vi "Acquire Data.vi"(0 "Data in":cluster{"Data":sgl[][]}[](array[cluster]), 1 "Trigger Index":i32, 5 "taskID":u32, 7 "Device Channel Lists":T11(array[cluster]), 9 "CJTEMP Chan Indexes":T12(array[cluster]), 11 "Channel Filter":bool[](array[boolean])) -> (4 "Data out":cluster{"Data":sgl[][]}[](array[cluster]), 6 "Acquiring Data":bool, 15 "error out":errorcluster)   [LabVIEW 2019]
uses:
  AI Read (waveform).vi
  AI Read (scaled array).vi
  <vilib>/measure/NI_MAPro.lvlib
  <vilib>/measure/mamon.llb/Trigger Detection for 1 Channel (obs).vi
  Type Defs and Controls/DAQ Settings.ctl
  Type Defs and Controls/Channel Config.ctl
  Type Defs and Controls/Header.ctl
  Type Defs and Controls/Sensor Config.ctl
  Type Defs and Controls/Trigger Stop Method.ctl
  Type Defs and Controls/Log File Type.ctl
  Type Defs and Controls/Graph Settings Type Def.ctl
  Type Defs and Controls/Test Limits.ctl
  Type Defs and Controls/Part Info.ctl
  Type Defs and Controls/All Part Info.ctl
panel:
  in  "taskID in":u32 format="%x"
  out "DAQ Active":bool
  in  "Data In":sgl[][](array[numeric])
  out "Data Out":sgl[][](array[numeric])
  out "DAQ Active out":bool
  in  "DAQ Active in":bool=TRUE
  in  "Config":T1={"DAQ Settings"={"Trigger Type"=enum."Manual", "Trigger Samples"=0, "Pretrigger Samples"=0, "Trigger Interval"=0.0, "Time Units"=FALSE, "Auto Save"=FALSE, "Sample Rate"=7.0, "Select Analog"=FALSE, "Trigger Value"=0.0, "Trigger Stop Method"=enum."Use Samples Value to Stop Trigger", "Rate Sec/Min"=FALSE, "Save Mode"=enum."Single File", "File Size Limit"=0.0, "Log File Type"=enum."Basic", "Trigger Data Index"=0}, "Channels"=[], "Header"={"TA Number"="", "Test Name"="", "Serial Number"="", "Technician"=""}, "Graph Settings"={"Graph Labels"=[], [], [], [], [], [], [], [], [], [], [], [], [], "Graph Toggles"=[], "Axis Toggles"=[], "Graph Range"=enum."1"}, "Test Limits"=[], "All Type Info"=[], "Save Mode"=enum."Single File"} {"DAQ Settings"."Trigger Interval" min=0.0; "DAQ Settings"."Pretrigger Samples" min=0; "DAQ Settings"."Trigger Samples" min=0}
  out "Data":sgl[][](array[numeric])
  # "EGU"
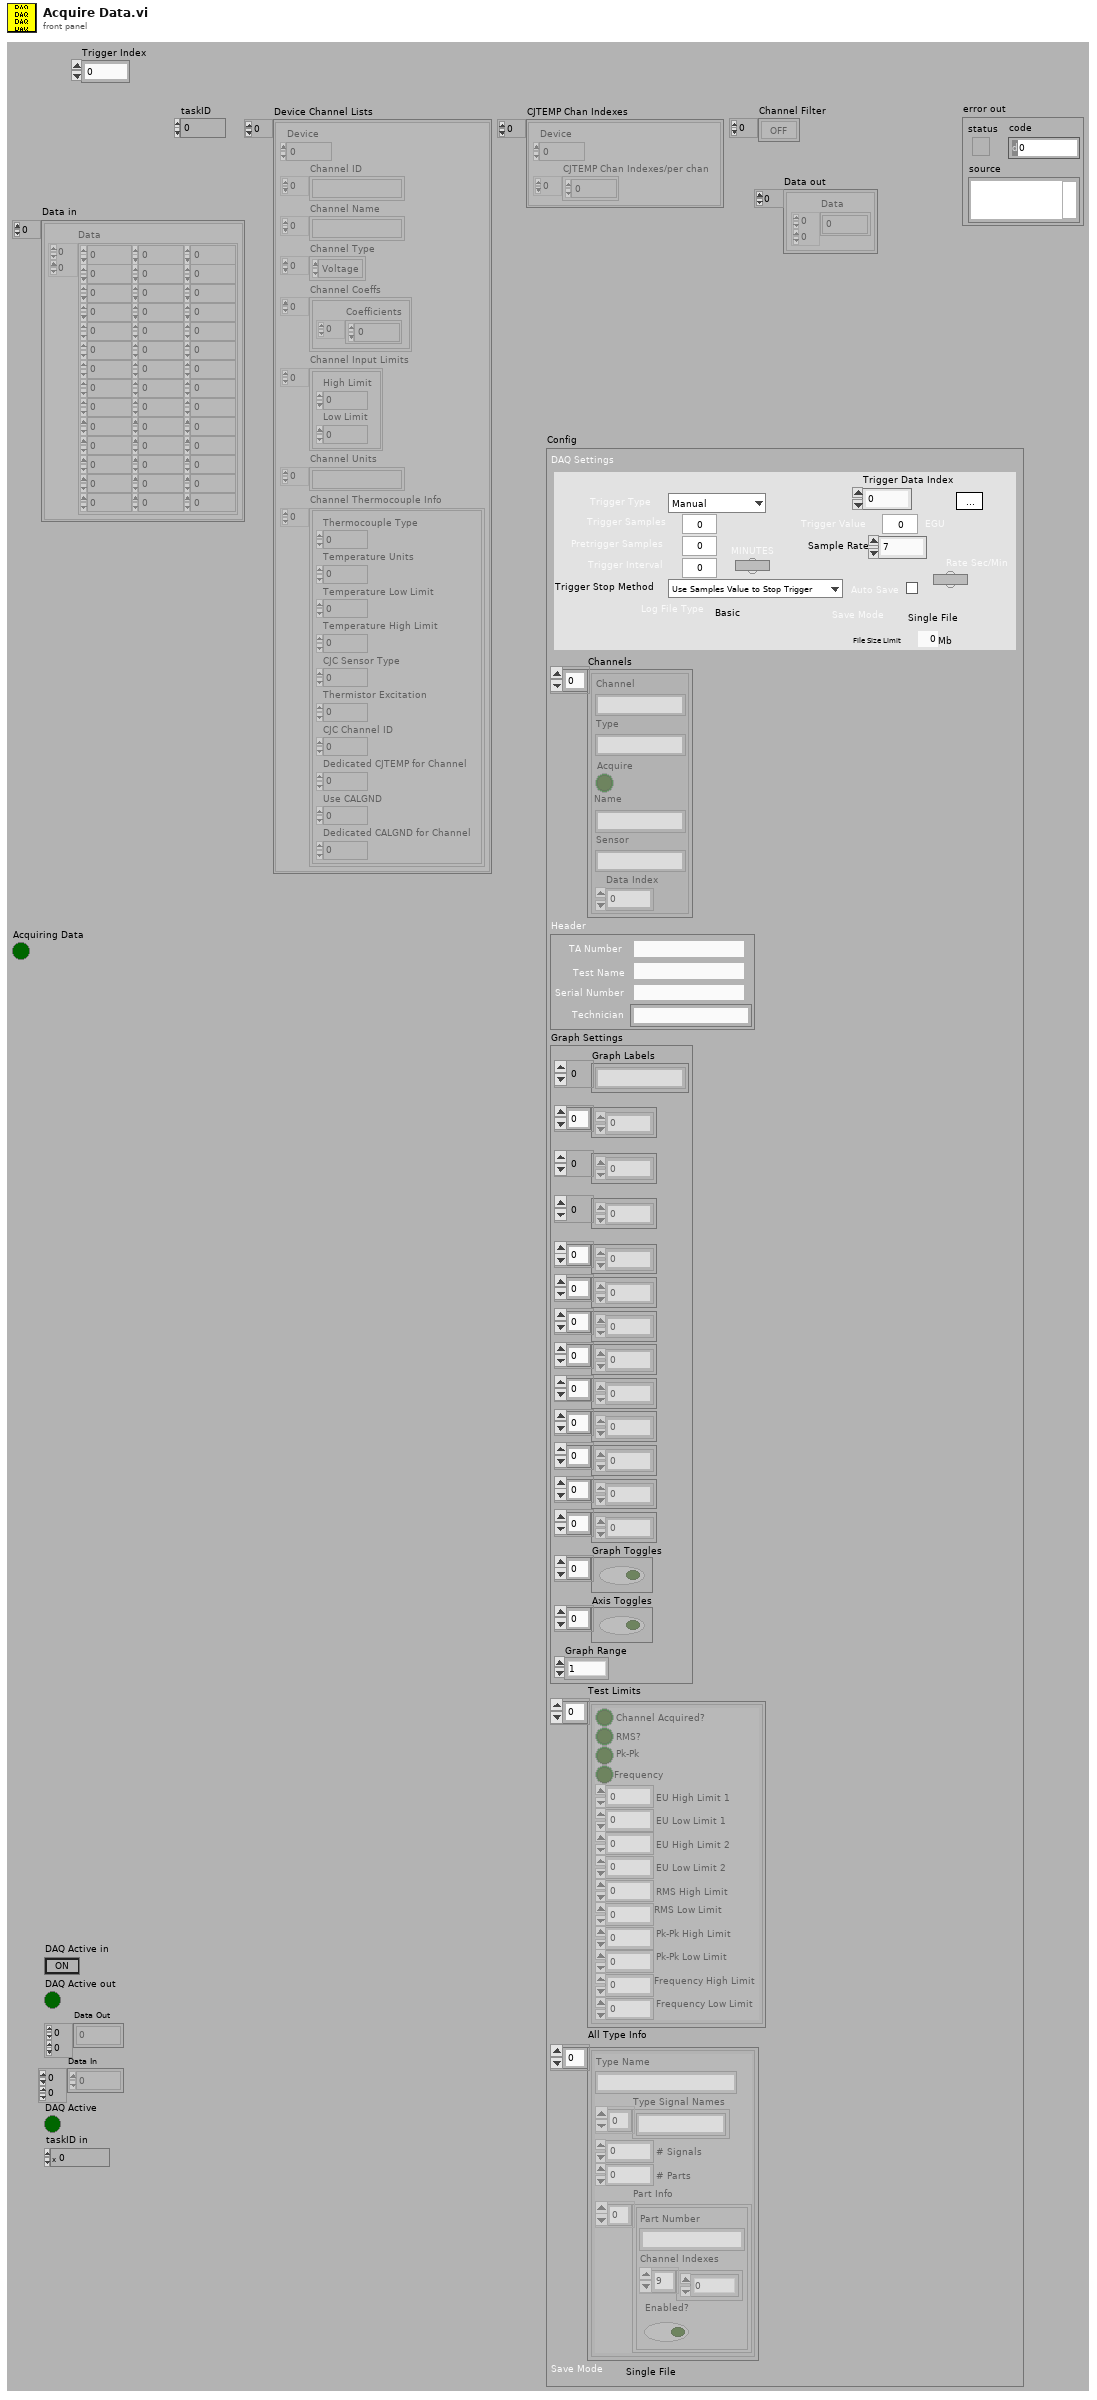
[diagram p1: front panel]
types:
  T1 = typedef "Sensor Config.ctl" = cluster{"DAQ Settings":T2, "Channels":T5[], "Header":T6, "Graph Settings":T7, "Test Limits":T8[], "All Type Info":T9, "Save Mode":enum16{"Single File", "Segmented Files", "New File at Midnight"}}
  T2 = typedef "DAQ Settings.ctl" = cluster{"Trigger Type":enum16{"Manual", "Timed", "Analog Rising", "Analog Falling"}, "Trigger Samples":i32, "Pretrigger Samples":i32, "Trigger Interval":dbl, "Time Units":bool, "Auto Save":bool, "Sample Rate":dbl, "Select Analog":bool, "Trigger Value":dbl, "Trigger Stop Method":T3, "Rate Sec/Min":bool, "Save Mode":enum16{"Single File", "Segmented Files", "New File at Midnight"}, "File Size Limit":dbl, "Log File Type":T4, "Trigger Data Index":u32}
  T3 = typedef "Trigger Stop Method.ctl" = enum16{"Use Samples Value to Stop Trigger", "Use Threshold to Stop Trigger"}
  T4 = typedef "Log File Type.ctl" = enum16{"Basic", "RTS"}
  T5 = typedef "Channel Config.ctl" = cluster{"Channel":string, "Type":string, "Acquire":bool, "Name":string, "Sensor":string, "Data Index":u32}
  T6 = typedef "Header.ctl" = cluster{"TA Number":string, "Test Name":string, "Serial Number":string, "Technician":string}
  T7 = typedef "Graph Settings Type Def.ctl" = cluster{"Graph Labels":string[], u8[], i16[], u32[], u8[], u8[], u8[], u32[], u8[], u8[], u8[], dbl[], dbl[], "Graph Toggles":bool[], "Axis Toggles":bool[], "Graph Range":enum16{"1", "2", "3", "4", "5", "10", "15", "30", "60"}}
  T8 = typedef "Test Limits.ctl" = cluster{"Channel Acquired?":bool, "RMS?":bool, "Pk-Pk":bool, "Frequency":bool, "EU High Limit 1":dbl, "EU Low Limit 1":dbl, "EU High Limit 2":dbl, "EU Low Limit 2":dbl, "RMS High Limit":dbl, "RMS Low Limit":dbl, "Pk-Pk High Limit ":dbl, "Pk-Pk Low Limit":dbl, "Frequency High Limit":dbl, "Frequency Low Limit":dbl}
  T9 = typedef "All Part Info.ctl" = cluster{"Type Name":string, "Type Signal Names":string[], "# Signals":i32, "# Parts":i32, "Part Info":T10[]}[]
  T10 = typedef "Part Info.ctl" = cluster{"Part Number":string, "Channel Indexes":u16[], "Enabled?":bool}
  T11 = cluster{"Device":i16, "Channel ID":string[], "Channel Name":string[], "Channel Type":enum16{"Voltage", "Thermocouple"}[], "Channel Coeffs":cluster{"Coefficients":dbl[]}[], "Channel Input Limits":cluster{"High Limit":dbl, "Low Limit":dbl}[], "Channel Units":string[], "Channel Thermocouple Info":cluster{"Thermocouple Type":u16, "Temperature Units":u16, "Temperature Low Limit":sgl, "Temperature High Limit":sgl, "CJC Sensor Type":u16, "Thermistor Excitation":u16, "CJC Channel ID":u16, "Dedicated CJTEMP for Channel":u16, "Use CALGND":u16, "Dedicated CALGND for Channel":u16}[]}[]
  T12 = cluster{"Device":i16, "CJTEMP Chan Indexes/per chan":i32[]}[]
  T13 = enum16{"Manual", "Timed", "Analog Rising", "Analog Falling"}
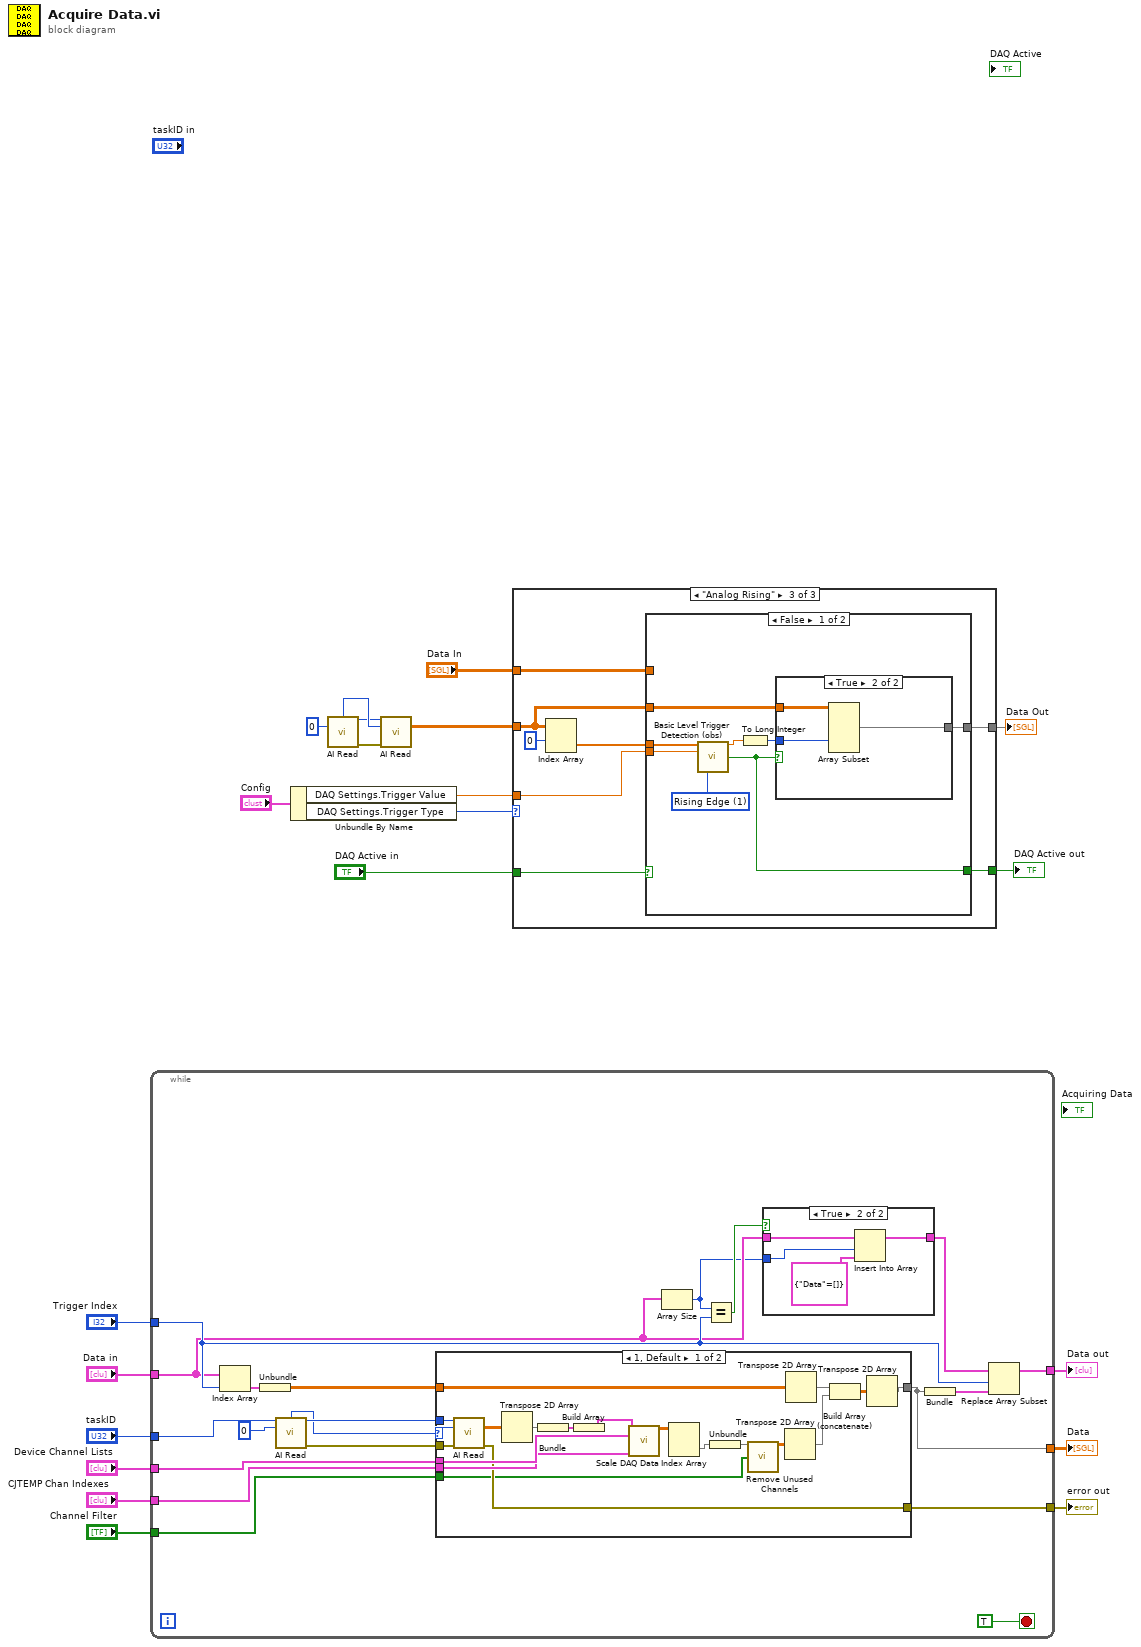
[diagram p0: block diagram]
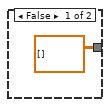
[diagram p4: hidden frame]
diagram:
  n1 = while {
    tunnel: [w41] -> w21
    tunnel: "Device Channel Lists" -> [w40]
    tunnel: "taskID" -> [w39]
    tunnel: "CJTEMP Chan Indexes" -> [w38]
    tunnel: "Channel Filter" -> [w37]
    tunnel: [w36] -> w16
    tunnel: [w35] -> w15
    tunnel: "Trigger Index" -> [w34]
    tunnel: "Data in" -> [w33]
    stop <- TRUE stop-if-true
    n2 = Index Array(array=w33, index=w34) -> (element=w29:cluster{"Data":sgl[][]})
    n3 = Unbundle(w29) -> ("Data"=w28:sgl[][])
    n4 = call-poly "AI Read.vi"("taskID in"=w39, "number of scans to read (-1:all)"=0) -> ("scan backlog"=w24:u32, "taskID out"=w30:u32, "error out"=w31:errorcluster)  [unwired: 8 in, 3 out]
    n5 = case shown="1, Default" w24 {
      selector: w24 -> [w57 _]
      tunnel: w30 -> [w66 _]
      tunnel: w31 -> [w65 _]
      tunnel: w40 -> [w61 _]
      tunnel: w38 -> [w60 _]
      tunnel: [w51 w67] -> w36
      tunnel: w28 -> [w54 w67]
      tunnel: [w56 _] -> w41
      tunnel: w37 -> [w47 _]
      frame 1, Default {
        n6 = call-poly "AI Read.vi"("taskID in"=w66, "number of scans to read (-1:all)"=w57, "error in (no error)"=w65) -> ("scaled data"=w64:sgl[][], "error out"=w56:errorcluster)  [unwired: 7 in, 4 out]
        n7 = Transpose 2D Array(2D array=w64) -> (transposed array=w50:sgl[][])
        n8 = Bundle(w50) -> (w63:cluster{sgl[][]})  [unwired: 1 in]
        n9 = Build Array(w63) -> (w62:cluster{sgl[][]}[])
        n10 = call "Scale DAQ Data.vi"("Data Read"=w62, "Coefficients"=w61, 11:w60) -> ("Scaled Data"=w59:sgl[][])  [unwired: 12 in]
        n11 = Index Array(array=w59) -> (element=w58:sgl[])  [unwired: 2 in]
        n12 = Unbundle(w58) -> (w49)
        n13 = call "Remove Unused Channels.vi"("Data in"=w49, "Channel Filter"=w47) -> ("Data out"=w48:sgl[][])  [unwired: 13 in]
        n14 = Transpose 2D Array(2D array=w48) -> (transposed array=w52:sgl[][])
        n15 = Transpose 2D Array(2D array=w54) -> (transposed array=w53:sgl[][])
        n16 = Build Array (concatenate)(w53, w52) -> (w55:sgl[][])
        n17 = Transpose 2D Array(2D array=w55) -> (transposed array=w51:sgl[][])
      }
      frame 0 {
      }
    }
    n18 = Array Size(array=w33) -> (size(s)=w25:i32)
    n19 = Equal?(x=w25, y=w34) -> (x = y?=w26:bool)
    n20 = case shown="True" w26 {
      tunnel: w33 -> [w42 w46]
      tunnel: w25 -> [_ w45]
      tunnel: [w42 w43] -> w22
      frame False {
      }
      frame True {
        n21 = Insert Into Array(array=w46, index=w45, new element=cluster{"Data":sgl[][]} {"Data"=[]} ("new element/subarray")) -> (w43:cluster{"Data":sgl[][]}[])
      }
    }
    n22 = Bundle("Data"=w36) -> (w27:cluster{"Data":sgl[][]})  [unwired: 1 in]
    n23 = Replace Array Subset(array=w22, new element=w27, index=w34) -> (w35:cluster{"Data":sgl[][]}[])
  }
  "error out" <- w21
  "Data out" <- w15
  "Data" <- w16
  n24 = Unbundle By Name("Config") -> ("DAQ Settings.Trigger Value"=w5:dbl, "DAQ Settings.Trigger Type"=w7:T13)
  n25 = call-poly "AI Read.vi"("number of scans to read (-1:all)"=0) -> ("scan backlog"=w10:u32, "taskID out"=w9:u32, "error out"=w8:errorcluster)  [unwired: 9 in, 3 out]
  n26 = call-poly "AI Read.vi"("taskID in"=w9, "number of scans to read (-1:all)"=w10, "error in (no error)"=w8) -> ("scaled data"=w6:sgl[][])  [unwired: 7 in, 5 out]
  n27 = case shown="\"Analog Rising\"" w7 {
    tunnel: w6 -> [_ _ w70]
    tunnel: w5 -> [_ _ w71]
    tunnel: "DAQ Active in" -> [_ _ w75]
    tunnel: [_ _ w74] -> w3
    tunnel: [_ _ w69] -> w2
    tunnel: "Data In" -> [_ _ w68]
    frame "Manual", Default {
    }
    frame "Timed" {
    }
    frame "Analog Rising" {
      n28 = Index Array(array=w70, index (row)=0) -> (element=w72:sgl[])  [unwired: 1 in]
      n29 = case shown="False" w75 {
        tunnel: [w80 _] -> w74
        tunnel: w72 -> [w83 _]
        tunnel: w71 -> [w82 _]
        tunnel: w70 -> [w79 _]
        tunnel: [w76 _] -> w69
        tunnel: w68 -> [_ _]
        frame False {
          w81 = u16 1 items=["Falling Edge", "Rising Edge"] ("slope")
          n30 = call-poly <vilib>:"Basic Level Trigger Detection (obs).vi"("signal in"=w83, "level"=w82, "trigger slope"=w81) -> ("trigger location"=w78:dbl, "trigger detected?"=w80:bool)  [unwired: 10 in, 1 out]
          n31 = To Long Integer(number=w78) -> (32bit integer=w77:i32)
          n32 = case shown="True" w80 {
            tunnel: w79 -> [_ w87]
            tunnel: w77 -> [_ w86]
            tunnel: [sgl[][] [] w85] -> w76
            frame False {
            }
            frame True {
              n33 = Array Subset(array=w87, index (col)=w86) -> (w85:sgl[][])  [unwired: 3 in]
            }
          }
        }
        frame True {
        }
      }
    }
  }
  "DAQ Active out" <- w3
  "Data Out" <- w2
